vi "自定义控件和枚举.vi"() -> ()   [LabVIEW 2023]
panel:
  out "Boolean":bool
  in  "stop":bool
  out "dropdown":i32
  in  "Ring":u16(ring) items=["Monday"=1, "Tuesday"=2, "Wendesday"=3, "Thursday"=4, "Friday"=5, "Saturday"=6, "Sunday"=7]
  out "Enum":i32
  in  "Enum":T1(ring)
  # "用户自定义控件与枚举"
  # "Enum 必须是从零开始的连续的 整数。  ring/dropdown 不是。 可以是任何数值，可以带符号。"
  # "选定图标， 然后 custome  然后一个状态 一个图标。"
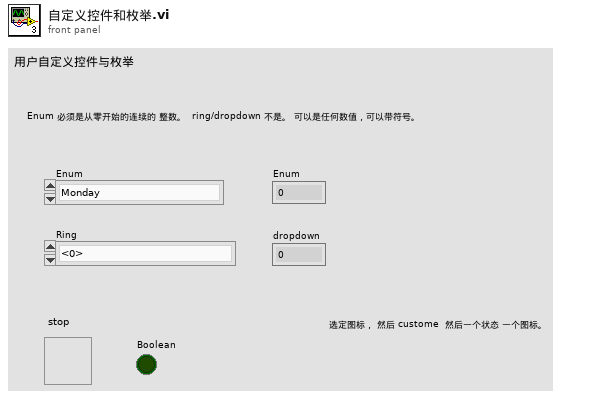
[diagram p1: front panel]
types:
  T1 = enum16{"Monday", "Tuesday ", "Wednesday", "Thursday", "Friday", "Saturday", "Sunday"}
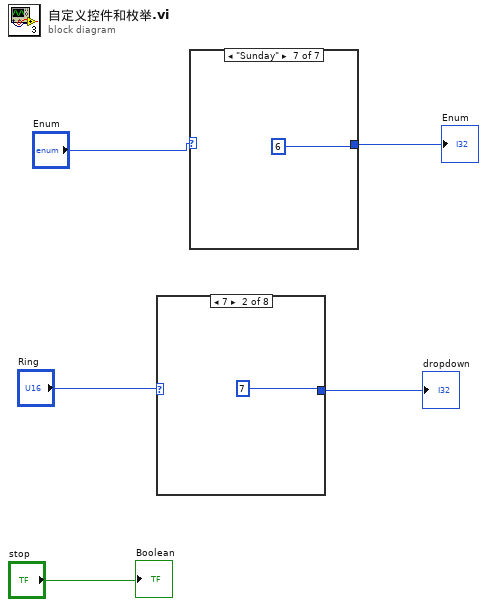
[diagram p0: block diagram]
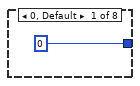
[diagram p2: hidden frame]
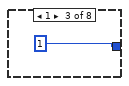
[diagram p3: hidden frame]
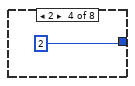
[diagram p4: hidden frame]
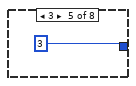
[diagram p5: hidden frame]
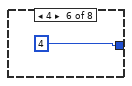
[diagram p6: hidden frame]
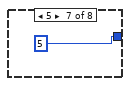
[diagram p7: hidden frame]
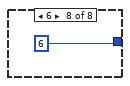
[diagram p8: hidden frame]
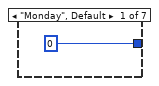
[diagram p9: hidden frame]
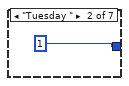
[diagram p10: hidden frame]
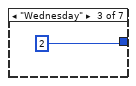
[diagram p11: hidden frame]
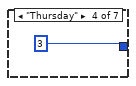
[diagram p12: hidden frame]
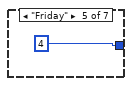
[diagram p13: hidden frame]
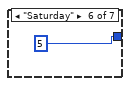
[diagram p14: hidden frame]
diagram:
  n1 = case shown="7" "Ring" {
    tunnel: [0 7 1 2 3 4 5 6] -> w2
    frame 0, Default {
    }
    frame 7 {
    }
    frame 1 {
    }
    frame 2 {
    }
    frame 3 {
    }
    frame 4 {
    }
    frame 5 {
    }
    frame 6 {
    }
  }
  "dropdown" <- w2
  n2 = case shown="\"Sunday\"" "Enum" {
    tunnel: [0 1 2 3 4 5 6] -> w4
    frame "Monday", Default {
    }
    frame "Tuesday " {
    }
    frame "Wednesday" {
    }
    frame "Thursday" {
    }
    frame "Friday" {
    }
    frame "Saturday" {
    }
    frame "Sunday" {
    }
  }
  "Enum" <- w4
  "Boolean" <- "stop"
